vi "Extreme Value Inverse CDF.vi"(9 "b":dbl=1.0, 10 "a":dbl, 11 "cdf(x)":dbl=0.5) -> (0 "error":i32, 3 "x":dbl=0.36651292058166435)   [LabVIEW 2020, in "NI_Gmath.lvlib"]
doc: "Computes the continuous inverse cumulative distribution function (CDF) of the various distributions. You must manually select the polymorphic instance to use."
uses:
  <vilib>/gmath/NI_Gmath.lvlib
  <vilib>/gmath/statdist.llb/st_error_code.ctl
panel:
  # "Extreme Value Inverse CDF"
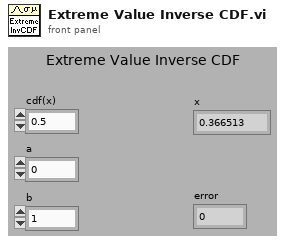
[diagram p1: front panel]
types:
  T1 = typedef "NI_Gmath.lvlib/st_error_code.ctl" = i32
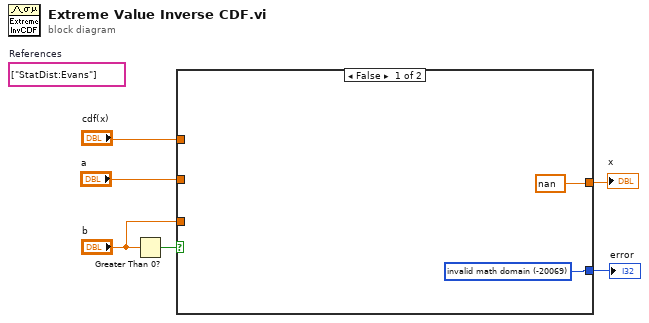
[diagram p0: block diagram]
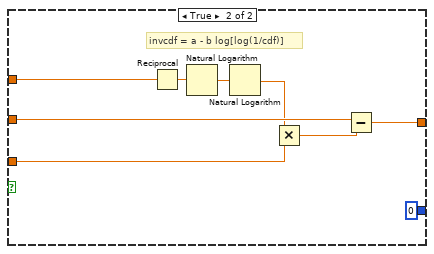
[diagram p2: hidden frame]
diagram:
  (unwired) string[] ["StatDist:Evans"]  # References
  n1 = Greater Than 0?(x="b") -> (x > 0?=w5:bool)
  n2 = case shown="False" w5 {
    tunnel: [w7 0 ("invalid math domain")] -> w1
    tunnel: [nan w9] -> w2
    tunnel: "a" -> [_ w16]
    tunnel: "b" -> [_ w12]
    tunnel: "cdf(x)" -> [_ w15]
    frame False {
      w7 = T1 -20069 items=["invalid math domain"=-20069, "Fourier interpolation size m >= n"=-20070, "empty array"=-20003] ("stat interp error code")
    }
    frame True {
      # "invcdf = a - b log[log(1/cdf)]"
      n3 = Reciprocal(x=w15) -> (1/x=w14:dbl)
      n4 = Natural Logarithm(1:w14) -> (0:w13:dbl)
      n5 = Natural Logarithm(1:w13) -> (0:w11:dbl)
      n6 = Multiply(x=w11, y=w12) -> (x*y=w10:dbl)
      n7 = Subtract(x=w16, y=w10) -> (x-y=w9:dbl)
    }
  }
  "x" <- w2
  "error" <- w1
